vi "Main Page.vi"(8 "error in (no error)":errorcluster, 11 "Node Ptr":T11 format="%.0x") -> (0 "error out":errorcluster)   [LabVIEW 2015, in "Chassis TimeSync System Explorer.lvlib"]
uses:
  Chassis TimeSync System Explorer.lvlib
  <vilib>/NI Veristand/Custom Device API/Custom Device Item Ref.ctl
  Connection Selection.ctl
  Shared/Routes.ctl
  Shared/Route.ctl
  Pins Tab.ctl
  Shared/Mode.ctl
  Shared/External Pin.ctl
  Shared/Time Reference.ctl
  Time Ref Tab.ctl
  Shared/IRIG Type.ctl
  <vilib>/NI Veristand/Custom Device API/Custom Device Channel Type.ctl
  Shared/Constants.vi
  <vilib>/NI Veristand/Custom Device API/Get Item Property (Boolean).vi
  sub_EnableDisable Control.vi
  <vilib>/NI Veristand/Custom Device API/Get Item Property (String).vi
  <vilib>/NI Veristand/Custom Device API/Get Item Property (U16).vi
  <vilib>/NI Veristand/Custom Device API/Get Item Property (Double).vi
  <vilib>/NI Veristand/Custom Device API/Set Item Property (String).vi
  <vilib>/NI Veristand/Custom Device API/Set Item Property (Boolean).vi
  <vilib>/NI Veristand/Custom Device API/Set Item Property (Variant).vi
  <vilib>/NI Veristand/Custom Device API/Set Item Property (U16).vi
  <vilib>/NI Veristand/Custom Device API/Set Item Property (I32).vi
  <vilib>/NI Veristand/Custom Device API/Set Item Property (Double).vi
  <vilib>/NI Veristand/Custom Device API/Custom Device API.lvlib
  Shared/Chassis TimeSync Shared.lvlib
panel:
  in  "6683H Warning":string
  in  "SyncModule":string caption="Chassis Clock Generation Module"
  in  "SyncModule?":bool
  in  "Settings":T1(tab)
  out "Mode Desciption":string
  in  "Mode":T2
  in  "ConSelection":T3 caption="Selection"
  out "Pins tab":T4
  in  "PFI2":bool
  in  "PFI1":bool
  in  "PFI0":bool
  in  "PXI_Trig0":bool
  in  "Route In Pin":T5
  in  "Custom Routes":T6
  out "TimeRefTab":T8
  in  "Priority 2":i32 min=0 max=255
  in  "Priority 1":i32 min=0 max=255
  in  "IRIG type":T9=enum."IRIGB AM"
  in  "Start Time":timestamp
  in  "PPSSetTime":bool
  in  "Terminal":string
  in  "Time Reference":T10
  out "Mode Desciption 2":string="When using a time reference other than PXI Backplane Clock, it is recommended to additionally configure that time refernece in Measurment and Automation Explorer (MAX) before deployment. Doing so will prevent \"macro\" adjustments to system time while the NI VeriStand engine is running."
  in  "StartDelay":u16 caption="Generation Start Delay (s)"
  in  "PhaseOffset":dbl caption="Generation Phase Offset (°)" min=0.0 max=360.0
  in  "timekeeper":string caption="Time-Based Synchronization Module"
  in  "Header":cluster{"Section Name":string}={"Section Name"="Chassis TimeSync Settings"}
  in  "Description":string
  in  "Name":string
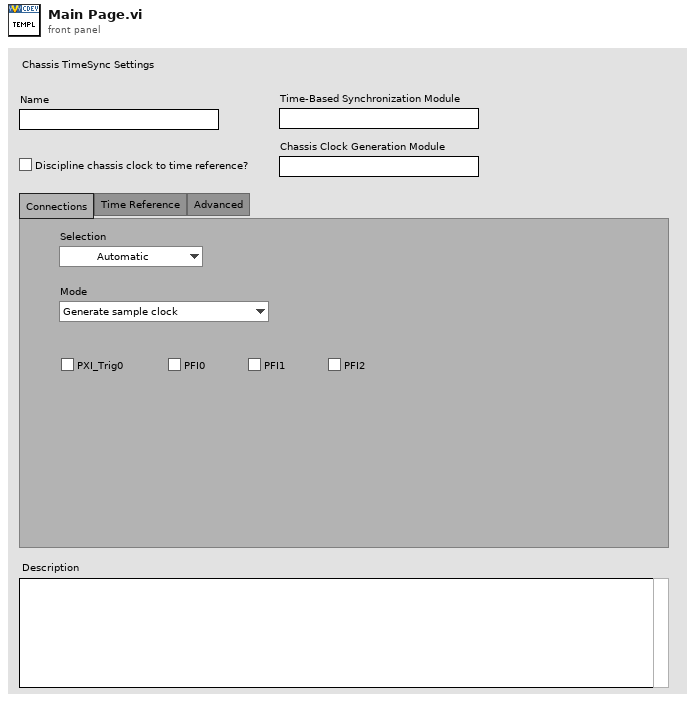
[diagram p1: front panel]
types:
  T1 = enum32{"Connections", "Time Reference", "Advanced"}
  T2 = typedef "Chassis TimeSync Shared.lvlib/Mode.ctl" = enum16{"Generate sample clock", "Route sample clock out of chassis", "Route sample clock into chassis", "Custom routes"}
  T3 = typedef "Chassis TimeSync System Explorer.lvlib/Connection Selection.ctl" = enum16{"Automatic", "Custom"}
  T4 = typedef "Chassis TimeSync System Explorer.lvlib/Pins Tab.ctl" = enum32{"Pins", "Ext. Pin", "Custom"}
  T5 = typedef "Chassis TimeSync Shared.lvlib/External Pin.ctl" = enum16{"PFI0", "PFI1", "PFI2"}
  T6 = typedef "Chassis TimeSync Shared.lvlib/Routes.ctl" = T7[]
  T7 = typedef "Chassis TimeSync Shared.lvlib/Route.ctl" = cluster{"Source":string, "Destination":string}
  T8 = typedef "Chassis TimeSync System Explorer.lvlib/Time Ref Tab.ctl" = enum32{"Empty", "1588", "IRIG", "PPS"}
  T9 = typedef "Chassis TimeSync Shared.lvlib/IRIG Type.ctl" = enum16{"IRIGB DC", "IRIGB AM"}
  T10 = typedef "Chassis TimeSync Shared.lvlib/Time Reference.ctl" = enum16{"GPS", "IRIG", "PPS", "1588 Ordinary Clock", "PXI Chassis Clock", "Free Running (Internal)"}
  T11 = typedef "Custom Device API.lvlib/Custom Device Item Ref.ctl" = u64
  T12 = typedef "Chassis TimeSync Shared.lvlib/Connection Settings.ctl" = cluster{"Mode":T2, "pxitrig":bool, "pfi0":bool, "pfi1":bool, "pfi2":bool, "External Pin":T5, "Routes":T6}
  T13 = typedef "Custom Device API.lvlib/Custom Device Item Info.ctl" = cluster{"Name":string, "Is Channel":bool, "GUID":string, "Is Waveform":bool}
  T14 = typedef "Chassis TimeSync Shared.lvlib/Time Ref Settings.ctl" = cluster{"Time Reference":T10, "Priority 1":i32, "Priority 2":i32, "IRIG type":T9, "Terminal":string, "PPSSetTime":bool, "Start Time":timestamp}
  T15 = typedef "Custom Device API.lvlib/Custom Device Channel Type.ctl" = enum16{"Input", "Output"}
  T16 = typedef "Custom Device API.lvlib/Custom Device Commands.ctl" = enum16{"Default", "Item renamed", "Shutdown", "Dynamic button pressed"}
  T17 = typedef "Chassis TimeSync Shared.lvlib/Channel.ctl" = cluster{"Name":string, "Units":string, "Default":dbl, "Description":string}
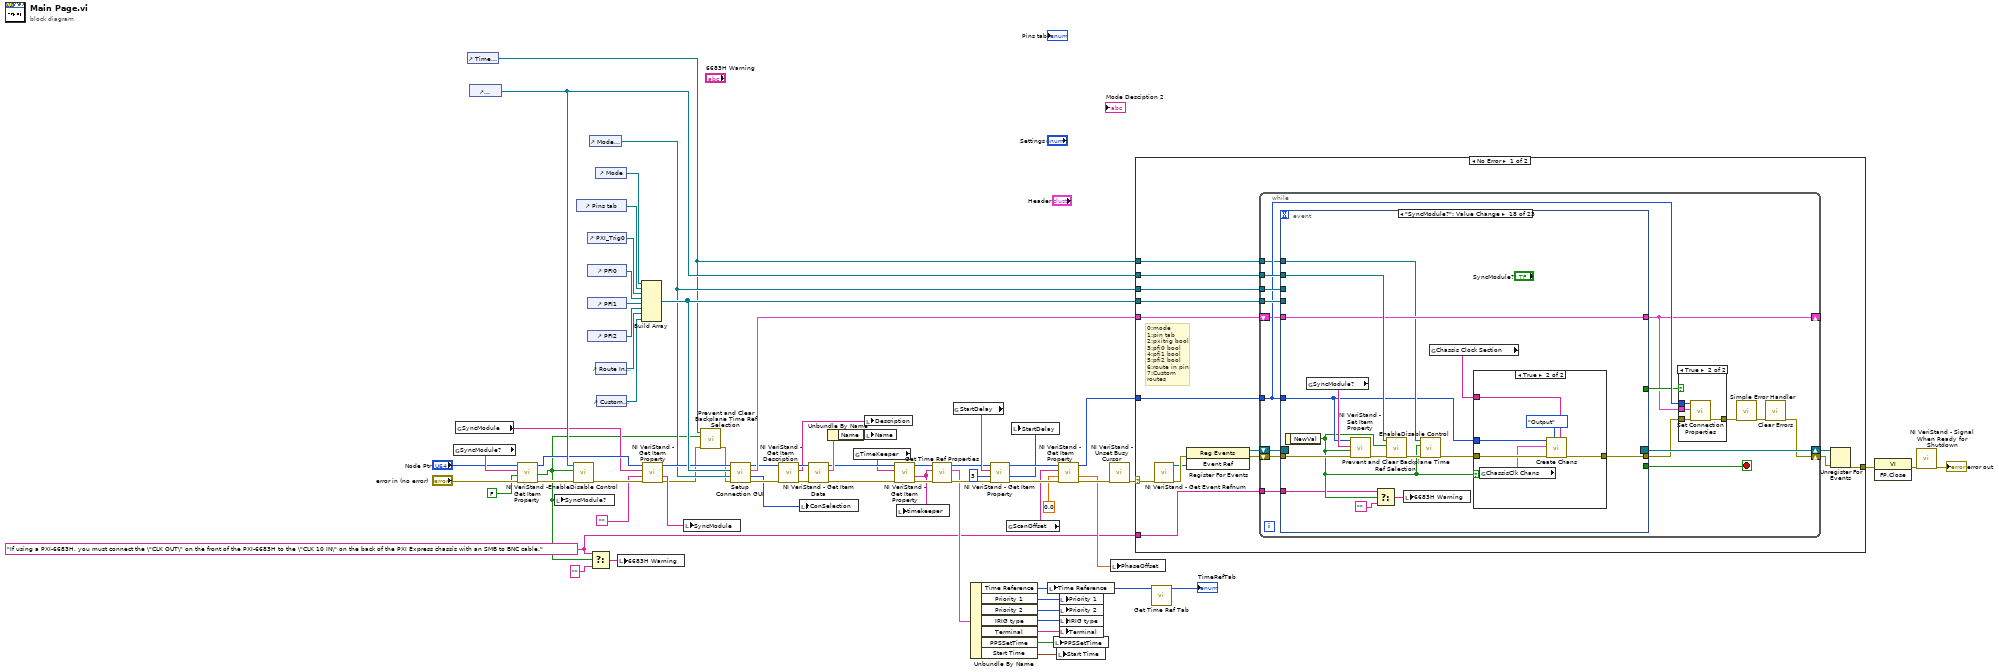
[diagram p0: block diagram]
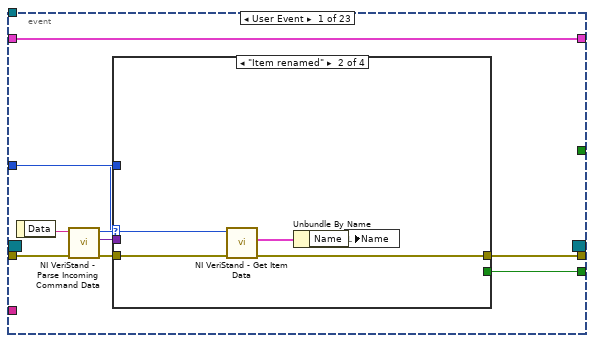
[diagram p3: hidden frame]
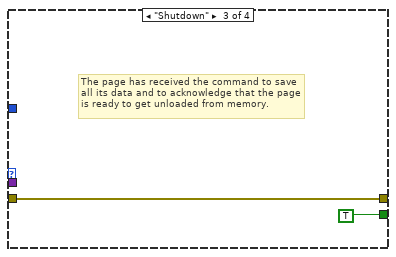
[diagram p5: hidden frame]
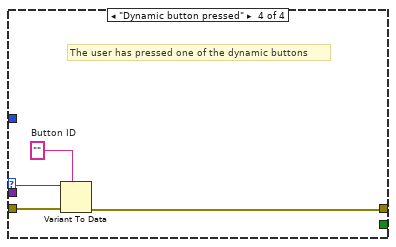
[diagram p6: hidden frame]
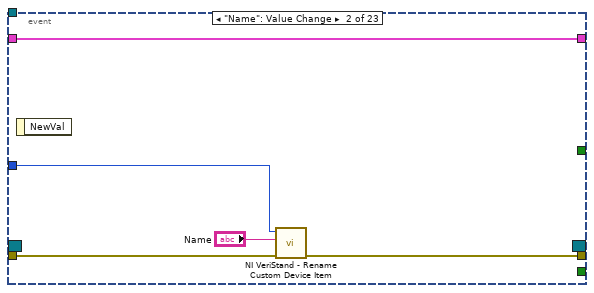
[diagram p7: hidden frame]
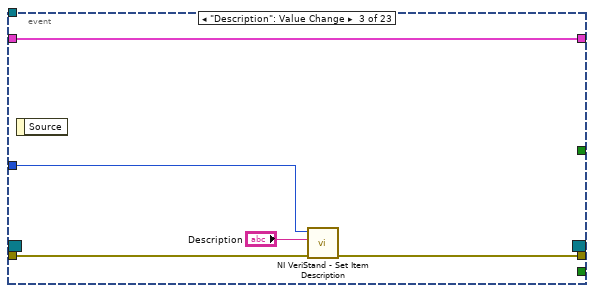
[diagram p8: hidden frame]
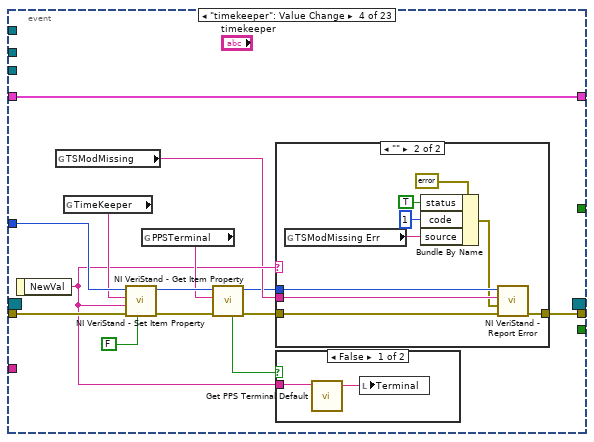
[diagram p9: hidden frame]
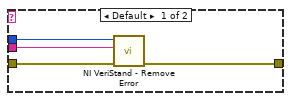
[diagram p10: hidden frame]
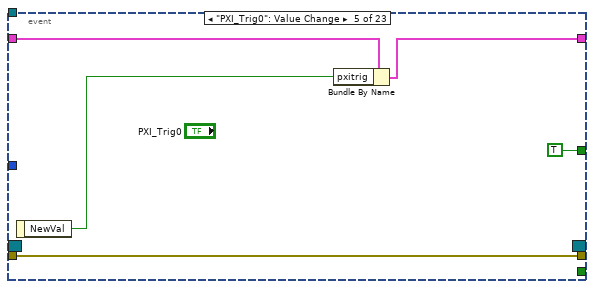
[diagram p12: hidden frame]
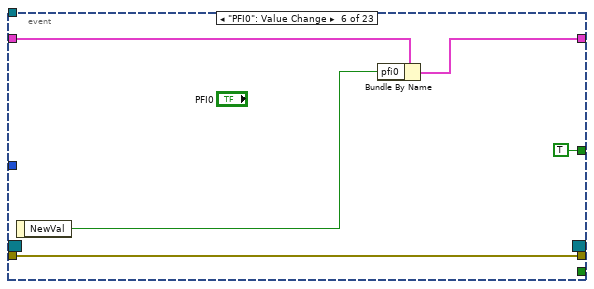
[diagram p13: hidden frame]
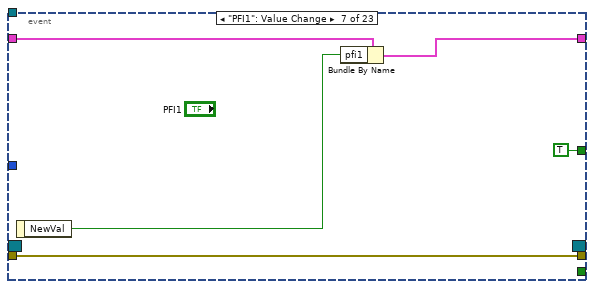
[diagram p14: hidden frame]
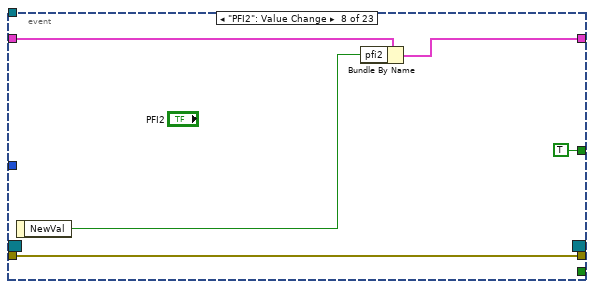
[diagram p15: hidden frame]
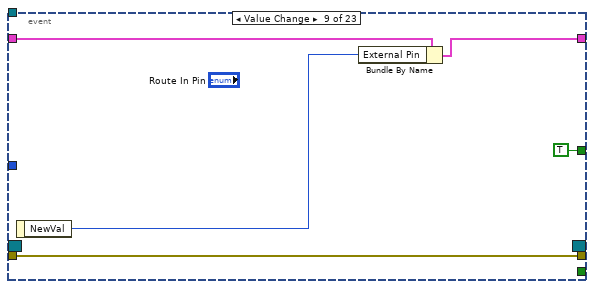
[diagram p16: hidden frame]
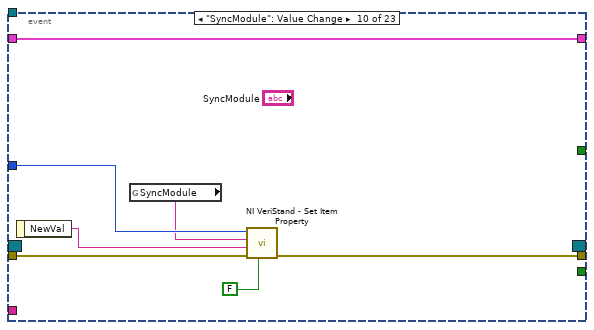
[diagram p17: hidden frame]
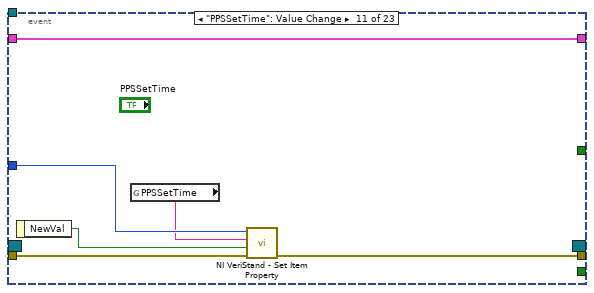
[diagram p18: hidden frame]
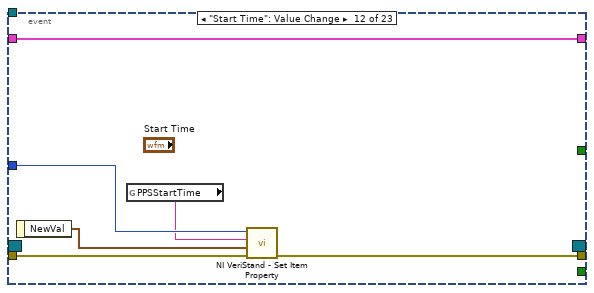
[diagram p19: hidden frame]
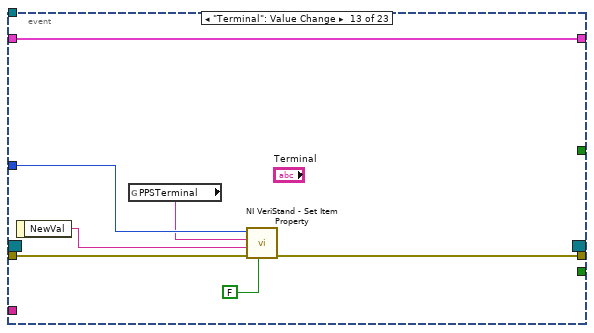
[diagram p20: hidden frame]
diagram:
  w1 = "If using a PXI-6683H, you must connect the \"CLK OUT\" on the front of the PXI-6683H to the \"CLK 10 IN\" on the back of the PXI Express chassis with an SMB to BNC cable." ("6683H Warning")
  n1 = global read "Constants.vi" "SyncModule?"() -> (w34:string)
  n2 = global read "Constants.vi" "SyncModule"() -> (w29:string)
  n3 = control-ref of="Time Reference"() -> (w7:refnum<vi>)
  n4 = control-ref of="SyncModule"() -> (w31:refnum<vi>)
  n5 = call-poly <vilib>:"NI VeriStand - Get Item Property.vi"("error in (no error)"="error in (no error)", "Default Value"=FALSE, "Property Name"=w34, "Item Ref in"="Node Ptr") -> ("error out"=w35:errorcluster, "Value"=w4:bool, "Item Ref out"=w30:T11)  [unwired: 4 in, 1 out]
  n6 = local write "SyncModule?"(w4) -> ()
  n7 = call-poly "EnableDisable Control.vi"("error in (no error)"=w35, "Enable"=w4, "Control"=w31) -> ("error out"=w32:errorcluster)  [unwired: 8 in]
  n8 = control-ref of="Pins tab"() -> (w45:refnum<vi>)
  n9 = control-ref of="PXI_Trig0"() -> (w44:refnum<vi>)
  n10 = control-ref of="PFI0"() -> (w43:refnum<vi>)
  n11 = control-ref of="PFI1"() -> (w38:refnum<vi>)
  n12 = control-ref of="PFI2"() -> (w39:refnum<vi>)
  n13 = control-ref of="Mode Desciption"() -> (w9:refnum<vi>)
  n14 = Select(t=w1, s=w4, f="" ("6683H Warning")) -> (s? t:f=w2:string)
  n15 = control-ref of="Mode"() -> (w46:refnum<vi>)
  n16 = control-ref of="Route In Pin"() -> (w42:refnum<vi>)
  n17 = control-ref of="Custom Routes"() -> (w41:refnum<vi>)
  n18 = local write "6683H Warning"(w2) -> ()
  n19 = Build Array(w46, w45, w44, w43, w38, w39, w42, w41) -> (w36:refnum<vi>[])
  n20 = call-poly <vilib>:"NI VeriStand - Get Item Property.vi"("error in (no error)"=w32, "Default Value"="", "Property Name"=w29, "Item Ref in"=w30) -> ("error out"=w6:errorcluster, "Value"=w27:string, "Item Ref out"=w10:T11)  [unwired: 4 in, 1 out]
  n21 = local write "SyncModule"(w27) -> ()
  n22 = call "Prevent and Clear Backplane Time Ref Selection.vi"("error in (no error)"=w6, "Sync Mod?"=w4, "Time Reference Enum"=w7) -> ("error out"=w5:errorcluster)  [unwired: 8 in]
  n23 = call "Setup Connection GUI.vi"("error in (no error)"=w5, "Mode Description Control"=w9, "Connection Controls"=w36, "Item Ref in"=w10) -> ("error out"=w37:errorcluster, "ConSelection"=w13:T3, "Connection Settings"=w12:T12, "Item Ref out"=w11:T11)  [unwired: 4 in]
  n24 = call <vilib>:"NI VeriStand - Get Item Description.vi"("error in (no error)"=w37, "Item Ref in"=w11) -> ("error out"=w63:errorcluster, "Description"=w64:string, "Item Ref out"=w65:T11)  [unwired: 7 out]
  n25 = local write "ConSelection"(w13) -> ()
  n26 = call <vilib>:"NI VeriStand - Get Item Data.vi"("error in (no error)"=w63, "Item Ref in"=w65) -> ("error out"=w60:errorcluster, "Item Info"=w62:T13, "Item Ref out"=w59:T11)  [unwired: 7 out]
  n27 = Unbundle By Name(w62) -> ("Name"=w61:string)
  n28 = global read "Constants.vi" "TimeKeeper"() -> (w58:string)
  n29 = local write "Description"(w64) -> ()
  n30 = local write "Name"(w61) -> ()
  n31 = call-poly <vilib>:"NI VeriStand - Get Item Property.vi"("error in (no error)"=w60, "Property Name"=w58, "Item Ref in"=w59) -> ("error out"=w57:errorcluster, "Value"=w23:string, "Item Ref out"=w25:T11)  [unwired: 5 in, 1 out]
  n32 = local write "timekeeper"(w23) -> ()
  n33 = call "Get Time Ref Properties.vi"("error in (no error)"=w57, "TimeKeeper Module"=w23, "Device Item Ref in"=w25) -> ("error out"=w26:errorcluster, "Time Ref Settings"=w22:T14, "Item Ref out"=w24:T11)  [unwired: 6 in]
  n34 = global read "Constants.vi" "StartDelay"() -> (w52:string)
  n35 = Unbundle By Name(w22) -> ("Time Reference"=w15:T10, "Priority 1"=w21:i32, "Priority 2"=w20:i32, "IRIG type"=w19:T9, "Terminal"=w18:string, "PPSSetTime"=w17:bool, "Start Time"=w16:timestamp)
  n36 = call-poly <vilib>:"NI VeriStand - Get Item Property.vi"("error in (no error)"=w26, "Default Value"=u16 3 ("Start Offset Multiple"), "Property Name"=w52, "Item Ref in"=w24) -> ("error out"=w53:errorcluster, "Value"=w50:u16, "Item Ref out"=w56:T11)  [unwired: 4 in, 1 out]
  n37 = global read "Constants.vi" "ScanOffset"() -> (w49:string)
  n38 = local write "StartDelay"(w50) -> ()
  n39 = local write "Time Reference"(w15) -> ()
  n40 = local write "PPSSetTime"(w17) -> ()
  n41 = local write "Start Time"(w16) -> ()
  n42 = call-poly <vilib>:"NI VeriStand - Get Item Property.vi"("error in (no error)"=w53, "Default Value"=0.0 ("Scan Offset Scale (%)"), "Property Name"=w49, "Item Ref in"=w56) -> ("error out"=w54:errorcluster, "Value"=w47:dbl, "Item Ref out"=w55:T11)  [unwired: 4 in, 1 out]
  n43 = local write "Priority 1"(w21) -> ()
  n44 = local write "Priority 2"(w20) -> ()
  n45 = local write "IRIG type"(w19) -> ()
  n46 = local write "Terminal"(w18) -> ()
  n47 = call <vilib>:"NI VeriStand - Unset Busy Cursor.vi"("error in (no error)"=w54) -> ("error out"=w66:errorcluster)  [unwired: 10 out]
  n48 = local write "PhaseOffset"(w47) -> ()
  n49 = case shown="No Error" w66 {
    selector: w66 -> [w76 w330]
    tunnel: [w81 w328] -> w69
    tunnel: w55 -> [w77 _]
    tunnel: w36 -> [w75 _]
    tunnel: w9 -> [w74 _]
    tunnel: w31 -> [w73 _]
    tunnel: w12 -> [w72 _]
    tunnel: w7 -> [w71 _]
    tunnel: w1 -> [w70 _]
    frame No Error {
      # "0:mode\n1:pin tab\n2:pxitrig bool\n3:pfi0 bool\n4:pfi1 bool\n5:pfi2 bool\n6:route in pin\n7:Custom routes"
      n50 = call <vilib>:"NI VeriStand - Get Event Refnum.vi"("error in (no error)"=w76) -> ("error out"=w84:errorcluster, "Event Ref"=w80:refnum<user-event>)  [unwired: 9 out]
      n51 = register-events(error in=w84, w80) -> (reference out=w78:refnum<event-registration>, error out=w79:errorcluster)  [unwired: 1 in]
      n52 = while {
        tunnel: w77 -> [w90]
        shift-right: [w96] -> w82
        shift-left: w79 -> [w100]
        shift-right: [w101] -> w83
        shift-left: w78 -> [w99]
        tunnel: w75 -> [w95]
        tunnel: w74 -> [w94]
        tunnel: w73 -> [w93]
        shift-right: [w86] -> _
        shift-left: w72 -> [w89]
        tunnel: w71 -> [w87]
        tunnel: w70 -> [w85]
        stop <- w98 stop-if-true
        n53 = event shown="[17] \"SyncModule?\": Value Change" {
          selector: w99 -> [_ _ _ _ _ _ _ _ _ _ _ _ _ _ _ _ _ _ _ _ _ _ _]
          dyn-events: [_ _ _ _ _ _ _ _ _ _ _ _ _ _ _ _ _ _ _ _ _ _ _] -> w101
          timeout: _ -> [_ _ _ _ _ _ _ _ _ _ _ _ _ _ _ _ _ _ _ _ _ _ _]
          tunnel: w100 -> [w115 w132 w136 w151 w171 w176 w181 w186 w191 w198 w204 w210 w217 w224 w230 w236 w242 w257 w275 w281 w287 w300 w323]
          tunnel: [w111 _ _ _ _ _ _ _ _ _ _ _ _ _ _ _ _ _ _ _ _ _ _] -> w98
          tunnel: [w110 w131 w135 w140 w171 w176 w181 w186 w191 w194 w200 w206 w213 w221 w226 w232 w238 w248 w275 w277 w283 w295 w320] -> w91
          tunnel: w90 -> [w109 w130 w137 w150 _ _ _ _ _ w197 w203 w209 w216 w223 w229 w235 w241 w249 _ w280 w286 w299 _]
          tunnel: w95 -> [_ _ _ _ _ _ _ _ _ _ _ _ _ _ _ _ _ _ _ _ _ w297 w321]
          tunnel: w94 -> [_ _ _ _ _ _ _ _ _ _ _ _ _ _ _ _ _ _ _ _ _ w296 _]
          tunnel: w93 -> [_ _ _ _ _ _ _ _ _ _ _ _ _ _ _ _ _ w254 _ _ _ _ _]
          tunnel: [w107 w128 w133 w148 w168 w174 w179 w184 w189 w193 w199 w205 w212 w220 w225 w231 w237 w253 w273 w276 w282 w288 w309] -> w86
          tunnel: w89 -> [w107 w128 w133 w148 w169 w175 w180 w185 w190 w193 w199 w205 w212 w220 w225 w231 w237 w253 w274 w276 w282 w290 w310]
          tunnel: [_ _ _ _ TRUE TRUE TRUE TRUE TRUE _ _ _ _ _ _ _ _ _ TRUE _ _ _ TRUE] -> w88
          tunnel: w87 -> [_ _ _ _ _ _ _ _ _ _ _ _ _ _ _ _ _ w252 _ _ _ _ _]
          tunnel: w85 -> [_ _ _ _ _ _ _ _ _ _ _ _ _ _ _ _ _ w245 _ _ _ _ _]
          event User Event {
            n54 = event-data() -> ("Data"=w114:string)  [unwired: 1 out]
            n55 = call <vilib>:"NI VeriStand - Parse Incoming Command Data.vi"("error in (no error)"=w115, "Incoming data"=w114) -> ("error out"=w113:errorcluster, "Outgoing data"=w108:variant, "Action"=w112:T16)  [unwired: 7 out]
            n56 = case shown="\"Item renamed\"" w112 {
              tunnel: w113 -> [w116 w121 w122 w127]
              tunnel: [_ _ TRUE _] -> w111
              tunnel: [w116 w118 w122 w124] -> w110
              tunnel: w109 -> [_ w120 _ _]
              tunnel: w108 -> [_ _ _ w126]
              frame "Default", Default {
              }
              frame "Item renamed" {
                n57 = call <vilib>:"NI VeriStand - Get Item Data.vi"("error in (no error)"=w121, "Item Ref in"=w120) -> ("error out"=w118:errorcluster, "Item Info"=w119:T13)  [unwired: 8 out]
                n58 = Unbundle By Name(w119) -> ("Name"=w117:string)
                n59 = local write "Name"(w117) -> ()
              }
              frame "Shutdown" {
                # "The page has received the command to save all its data and to acknowledge that the page is ready to get unloaded from memory."
              }
              frame "Dynamic button pressed" {
                w125 = ""  # Button ID
                # "The user has pressed one of the dynamic buttons"
                n60 = Variant To Data(error in=w127, type=w125, Variant=w126) -> (error out=w124:errorcluster)  [unwired: 1 out]
              }
            }
          }
          event "Name": Value Change {
            n61 = event-data() -> ()  [unwired: 2 out]
            n62 = call <vilib>:"NI VeriStand - Rename Custom Device Item.vi"("error in (no error)"=w132, "New Name"="Name", "Item Ref in"=w130) -> ("error out"=w131:errorcluster)  [unwired: 1 in, 7 out]
          }
          event "Description": Value Change {
            n63 = event-data() -> ()  [unwired: 2 out]
            n64 = call <vilib>:"NI VeriStand - Set Item Description.vi"("error in (no error)"=w136, "Description"="Description", "Item Ref in"=w137) -> ("error out"=w135:errorcluster)  [unwired: 8 out]
          }
          event "timekeeper": Value Change {
            n65 = event-data() -> ("NewVal"=w141:string)  [unwired: 1 out]
            n66 = global read "Constants.vi" "TSModMissing"() -> (w139:string)
            n67 = global read "Constants.vi" "TimeKeeper"() -> (w149:string)
            n68 = call-poly <vilib>:"NI VeriStand - Set Item Property.vi"("Binary String (T)"=FALSE, "error in (no error)"=w151, "Value"=w141, "Property Name"=w149, "Item Ref in"=w150) -> ("error out"=w146:errorcluster, "Item Ref out"=w145:T11)  [unwired: 4 in, 1 out]
            n69 = global read "Constants.vi" "PPSTerminal"() -> (w144:string)
            n70 = call-poly <vilib>:"NI VeriStand - Get Item Property.vi"("error in (no error)"=w146, "Property Name"=w144, "Item Ref in"=w145) -> ("error out"=w142:errorcluster, "Item Ref out"=w138:T11, "Found?"=w143:bool)  [unwired: 5 in, 1 out]
            n71 = case shown="\"\"" w141 {
              tunnel: w142 -> [w155 w164]
              tunnel: [w152 w163] -> w140
              tunnel: w139 -> [w154 w162]
              tunnel: w138 -> [w153 w161]
              frame Default {
                n72 = call <vilib>:"NI VeriStand - Remove Error.vi"("error in (no error)"=w155, "Error ID"=w154, "Node Ref in"=w153) -> ("error out"=w152:errorcluster)  [unwired: 7 in, 1 out]
              }
              frame "" {
                n73 = global read "Constants.vi" "TSModMissing Err"() -> (w157:string)
                n74 = Bundle By Name(cluster=errorcluster {"status"=FALSE, "code"=0, "source"=""} ("error constant"), "status"=TRUE, "code"=1, "source"=w157) -> (w156:errorcluster)
                n75 = call <vilib>:"NI VeriStand - Report Error.vi"("error in (no error)"=w164, "New Error"=w156, "Error ID"=w162, "Node Ref in"=w161) -> ("error out"=w163:errorcluster)  [unwired: 6 in, 1 out]
              }
            }
            n76 = case shown="False" w143 {
              tunnel: w141 -> [w166 _]
              frame False {
                n77 = call "Get PPS Terminal Default.vi"("TimeKeeper Module"=w166) -> ("PPSTerminal Default"=w165:string)  [unwired: 10 in]
                n78 = local write "Terminal"(w165) -> ()
              }
              frame True {
              }
            }
          }
          event "PXI_Trig0": Value Change {
            n79 = event-data() -> ("NewVal"=w170:bool)  [unwired: 1 out]
            n80 = Bundle By Name(cluster=w169, "pxitrig"=w170) -> (w168:T12)
          }
          event "PFI0": Value Change {
            n81 = event-data() -> ("NewVal"=w173:bool)  [unwired: 1 out]
            n82 = Bundle By Name(cluster=w175, "pfi0"=w173) -> (w174:T12)
          }
          event "PFI1": Value Change {
            n83 = event-data() -> ("NewVal"=w178:bool)  [unwired: 1 out]
            n84 = Bundle By Name(cluster=w180, "pfi1"=w178) -> (w179:T12)
          }
          event "PFI2": Value Change {
            n85 = event-data() -> ("NewVal"=w183:bool)  [unwired: 1 out]
            n86 = Bundle By Name(cluster=w185, "pfi2"=w183) -> (w184:T12)
          }
          event Value Change {
            n87 = event-data() -> ("NewVal"=w188:T5)  [unwired: 1 out]
            n88 = Bundle By Name(cluster=w190, "External Pin"=w188) -> (w189:T12)
          }
          event "SyncModule": Value Change {
            n89 = event-data() -> ("NewVal"=w195:string)  [unwired: 1 out]
            n90 = global read "Constants.vi" "SyncModule"() -> (w196:string)
            n91 = call-poly <vilib>:"NI VeriStand - Set Item Property.vi"("Binary String (T)"=FALSE, "error in (no error)"=w198, "Value"=w195, "Property Name"=w196, "Item Ref in"=w197) -> ("error out"=w194:errorcluster)  [unwired: 4 in, 2 out]
          }
          event "PPSSetTime": Value Change {
            n92 = event-data() -> ("NewVal"=w201:bool)  [unwired: 1 out]
            n93 = global read "Constants.vi" "PPSSetTime"() -> (w202:string)
            n94 = call-poly <vilib>:"NI VeriStand - Set Item Property.vi"("error in (no error)"=w204, "Value"=w201, "Property Name"=w202, "Item Ref in"=w203) -> ("error out"=w200:errorcluster)  [unwired: 5 in, 2 out]
          }
          event "Start Time": Value Change {
            n95 = event-data() -> ("NewVal"=w207:timestamp)  [unwired: 1 out]
            n96 = global read "Constants.vi" "PPSStartTime"() -> (w208:string)
            n97 = call-poly <vilib>:"NI VeriStand - Set Item Property.vi"("error in (no error)"=w210, "Value"=w207, "Property Name"=w208, "Item Ref in"=w209) -> ("error out"=w206:errorcluster)  [unwired: 5 in, 2 out]
          }
          event "Terminal": Value Change {
            n98 = event-data() -> ("NewVal"=w214:string)  [unwired: 1 out]
            n99 = global read "Constants.vi" "PPSTerminal"() -> (w215:string)
            n100 = call-poly <vilib>:"NI VeriStand - Set Item Property.vi"("Binary String (T)"=FALSE, "error in (no error)"=w217, "Value"=w214, "Property Name"=w215, "Item Ref in"=w216) -> ("error out"=w213:errorcluster)  [unwired: 4 in, 2 out]
          }
          event Value Change {
            n101 = event-data() -> ("NewVal"=w219:T10)  [unwired: 1 out]
            n102 = call "Get Time Ref Tab.vi"("Time Ref"=w219) -> ("TimeRefTab"=w218:T8)  [unwired: 10 in]
            n103 = global read "Constants.vi" "TimeRef"() -> (w222:string)
            n104 = local write "TimeRefTab"(w218) -> ()
            n105 = call-poly <vilib>:"NI VeriStand - Set Item Property.vi"("error in (no error)"=w224, "Value"=w219, "Property Name"=w222, "Item Ref in"=w223) -> ("error out"=w221:errorcluster)  [unwired: 5 in, 2 out]
          }
          event Value Change {
            n106 = event-data() -> ("NewVal"=w227:T9)  [unwired: 1 out]
            n107 = global read "Constants.vi" "IRIGType"() -> (w228:string)
            n108 = call-poly <vilib>:"NI VeriStand - Set Item Property.vi"("error in (no error)"=w230, "Value"=w227, "Property Name"=w228, "Item Ref in"=w229) -> ("error out"=w226:errorcluster)  [unwired: 5 in, 2 out]
          }
          event "Priority 1": Value Change {
            n109 = event-data() -> ("NewVal"=w233:i32)  [unwired: 1 out]
            n110 = global read "Constants.vi" "Priority1"() -> (w234:string)
            n111 = call-poly <vilib>:"NI VeriStand - Set Item Property.vi"("error in (no error)"=w236, "Value"=w233, "Property Name"=w234, "Item Ref in"=w235) -> ("error out"=w232:errorcluster)  [unwired: 5 in, 2 out]
          }
          event "Priority 2": Value Change {
            n112 = event-data() -> ("NewVal"=w239:i32)  [unwired: 1 out]
            n113 = global read "Constants.vi" "Priority2"() -> (w240:string)
            n114 = call-poly <vilib>:"NI VeriStand - Set Item Property.vi"("error in (no error)"=w242, "Value"=w239, "Property Name"=w240, "Item Ref in"=w241) -> ("error out"=w238:errorcluster)  [unwired: 5 in, 2 out]
          }
          event "SyncModule?": Value Change {
            n115 = event-data() -> ("NewVal"=w246:bool)  [unwired: 1 out]
            n116 = global read "Constants.vi" "SyncModule?"() -> (w256:string)
            n117 = call-poly <vilib>:"NI VeriStand - Set Item Property.vi"("error in (no error)"=w257, "Value"=w246, "Property Name"=w256, "Item Ref in"=w249) -> ("error out"=w255:errorcluster)  [unwired: 5 in, 2 out]
            n118 = Select(t=w245, s=w246, f="") -> (s? t:f=w243:string)
            n119 = call-poly "EnableDisable Control.vi"("error in (no error)"=w255, "Enable"=w246, "Control"=w254) -> ("error out"=w251:errorcluster)  [unwired: 8 in]
            n120 = local write "6683H Warning"(w243) -> ()
            n121 = call "Prevent and Clear Backplane Time Ref Selection.vi"("error in (no error)"=w251, "Sync Mod?"=w246, "Time Reference Enum"=w252) -> ("error out"=w250:errorcluster)  [unwired: 8 in]
            n122 = global read "Constants.vi" "Chassis Clock Section"() -> (w247:string)
            n123 = case shown="True" w246 {
              tunnel: w250 -> [w264 w270]
              tunnel: w249 -> [w263 w269]
              tunnel: [w258 w266] -> w248
              tunnel: w247 -> [w262 w265]
              frame False {
                n124 = call <vilib>:"NI VeriStand - Get Item Reference by Name.vi"("error in (no error)"=w264, "Item Name"=w262, "Parent Ref in"=w263) -> ("error out"=w261:errorcluster, "Item Ref"=w260:T11)  [unwired: 5 in, 2 out]
                n125 = call <vilib>:"NI VeriStand - Remove Custom Device Item.vi"("error in (no error)"=w261, "Force Delete (F)"=TRUE, "Item Ref in"=w260) -> ("error out"=w258:errorcluster)  [unwired: 7 in, 1 out]
              }
              frame True {
                n126 = global read "Constants.vi" "ChassisClk Chans"() -> (w267:T17[])
                n127 = call "Create Chans.vi"("New Section Name (none)"=w265, "Type"=Custom_Device_Channel_Type."Output", "error in (no error)"=w270, "Channels"=w267, "Section Ptr"=w269) -> ("error out"=w266:errorcluster)  [unwired: 5 in, 1 out]
              }
            }
          }
          event Value Change {
            n128 = event-data() -> ("NewVal"=w272:T6)  [unwired: 1 out]
            n129 = Bundle By Name(cluster=w274, "Routes"=w272) -> (w273:T12)
          }
          event "PhaseOffset": Value Change {
            n130 = event-data() -> ("NewVal"=w278:dbl)  [unwired: 1 out]
            n131 = global read "Constants.vi" "ScanOffset"() -> (w279:string)
            n132 = call-poly <vilib>:"NI VeriStand - Set Item Property.vi"("error in (no error)"=w281, "Value"=w278, "Property Name"=w279, "Item Ref in"=w280) -> ("error out"=w277:errorcluster)  [unwired: 5 in, 2 out]
          }
          event "StartDelay": Value Change {
            n133 = event-data() -> ("NewVal"=w284:u16)  [unwired: 1 out]
            n134 = global read "Constants.vi" "StartDelay"() -> (w285:string)
            n135 = call-poly <vilib>:"NI VeriStand - Set Item Property.vi"("error in (no error)"=w287, "Value"=w284, "Property Name"=w285, "Item Ref in"=w286) -> ("error out"=w283:errorcluster)  [unwired: 5 in, 2 out]
          }
          event Value Change {
            n136 = event-data() -> ("NewVal"=w293:T3)  [unwired: 1 out]
            n137 = global read "Constants.vi" "ConSelection"() -> (w298:string)
            n138 = call-poly <vilib>:"NI VeriStand - Set Item Property.vi"("error in (no error)"=w300, "Value"=w293, "Property Name"=w298, "Item Ref in"=w299) -> ("error out"=w294:errorcluster, "Item Ref out"=w291:T11)  [unwired: 5 in, 1 out]
            n139 = case shown="\"Custom\"" w293 {
              tunnel: w294 -> [w302 w307]
              tunnel: [w302 w306] -> w292
              tunnel: w291 -> [w301 w305]
              tunnel: w290 -> [_ w304]
              tunnel: [w301 w303] -> w289
              frame "Automatic" {
              }
              frame "Custom" {
                n140 = call "Set Connection Properties.vi"("error in (no error)"=w307, "AutoSelect"=w304, "Device Item Ref in"=w305) -> ("error out"=w306:errorcluster, "Item Ref out"=w303:T11)  [unwired: 7 in]
              }
            }
            n141 = call "Setup Connection GUI.vi"("error in (no error)"=w292, "Mode Description Control"=w296, "Connection Controls"=w297, "Item Ref in"=w289) -> ("error out"=w295:errorcluster, "Connection Settings"=w288:T12)  [unwired: 4 in, 2 out]
          }
          event Value Change {
            n142 = event-data() -> ("NewVal"=w313:T2)  [unwired: 1 out]
            n143 = Equal?(x=w313, y=Mode."Route sample clock out of chassis" ("x")) -> (x = y?=w311:bool)
            n144 = Equal?(x=w313, y=Mode."Generate sample clock" ("x")) -> (x = y?=w315:bool)
            n145 = Index Array(array=w321, index=2) -> (element=w317:refnum<vi>)
            n146 = call "Get Connection Description Text and Pins Tab.vi"("Mode"=w313) -> ("Pins tab"=w319:T4, "Description"=→"Mode Desciption":string)  [unwired: 9 in]
            n147 = local write "Pins tab"(w319) -> ()
            n148 = call-poly "EnableDisable Control.vi"("error in (no error)"=w323, "Enable"=w315, "Control"=w317) -> ("error out"=w320:errorcluster)  [unwired: 8 in]
            n149 = Bundle By Name(cluster=w310, "Mode"=w313) -> (w308:T12)
            n150 = case shown="True" w311 {
              tunnel: w308 -> [w324 w327]
              tunnel: [w324 w326] -> w309
              frame False {
              }
              frame True {
                n151 = Bundle By Name(cluster=w327, "pxitrig"=FALSE) -> (w326:T12)
              }
            }
          }
        }
        n152 = case shown="True" w88 {
          tunnel: [w102 w106] -> w92
          tunnel: w91 -> [w102 w105]
          tunnel: w90 -> [_ w104]
          tunnel: w86 -> [_ w103]
          frame False {
          }
          frame True {
            n153 = call "Set Connection Properties.vi"("error in (no error)"=w105, "AutoSelect"=w103, "Device Item Ref in"=w104) -> ("error out"=w106:errorcluster)  [unwired: 7 in, 1 out]
          }
        }
        n154 = call <vilib>:"Simple Error Handler.vi"("error in (no error)"=w92) -> ("error out"=w97:errorcluster)  [unwired: 1 in, 7 out]
        n155 = call <vilib>:"Clear Errors.vi"("error in (no error)"=w97) -> ("error out"=w96:errorcluster)  [unwired: 1 in, 5 out]
      }
      n156 = Unregister For Events(event registration refnum=w83, error in=w82) -> (error out=w81:errorcluster)
    }
    frame Error {
      n157 = call <vilib>:"Simple Error Handler.vi"("error in (no error)"=w330) -> ("error out"=w329:errorcluster)  [unwired: 1 in, 7 out]
      n158 = call <vilib>:"Clear Errors.vi"("error in (no error)"=w329) -> ("error out"=w328:errorcluster)  [unwired: 1 in, 5 out]
    }
  }
  n159 = call "Get Time Ref Tab.vi"("Time Ref"=w15) -> ("TimeRefTab"=→"TimeRefTab":T8)  [unwired: 10 in]
  n160 = invoke class="VI" method="FP.Close"(error in=w69) -> (error out=w68:errorcluster)  [unwired: 2 in, 2 out]
  n161 = call <vilib>:"NI VeriStand - Signal When Ready for Shutdown.vi"("error in (no error)"=w68) -> ("error out"=→"error out":errorcluster)  [unwired: 10 out]
